vi "Answer Eval.vi"(6 "Error Deviation (%)":dbl=5.0 format="%#_13g", 7 "Exercise Number":T1, 8 "error in":errorcluster, 9 "Waveform In":waveform(dbl), 11 "Exercise Folder Path":path) -> (0 "error out":errorcluster, 1 "Waveform Out":waveform(dbl)(graph), 2 "Response Array":bool[](array[boolean]), 3 "path":path)   [LabVIEW 2014]
uses:
  Ctls/ExerciseNumeration.ctl
  <vilib>/Analysis/baseanly.llb/Mean (DBL).vi
  <vilib>/express/express analysis/Spectral/Block/exnSpectralBlock spectral measurements peak poly.vi
  <vilib>/express/express analysis/Spectral/Block/exnSpectralBlock spectral measurements peak WFM.vi
  <vilib>/express/express analysis/Spectral/XNode/ExpressSpectralMeasurementsBlockNode.xnode
  <vilib>/Analysis/NI_AAL_SigProc.lvlib
  <vilib>/Analysis/NI_AALBase.lvlib
panel:
  out "Waveform In FFT":cluster{"f0":dbl, "df":dbl, "magnitude":dbl[]}(graph)
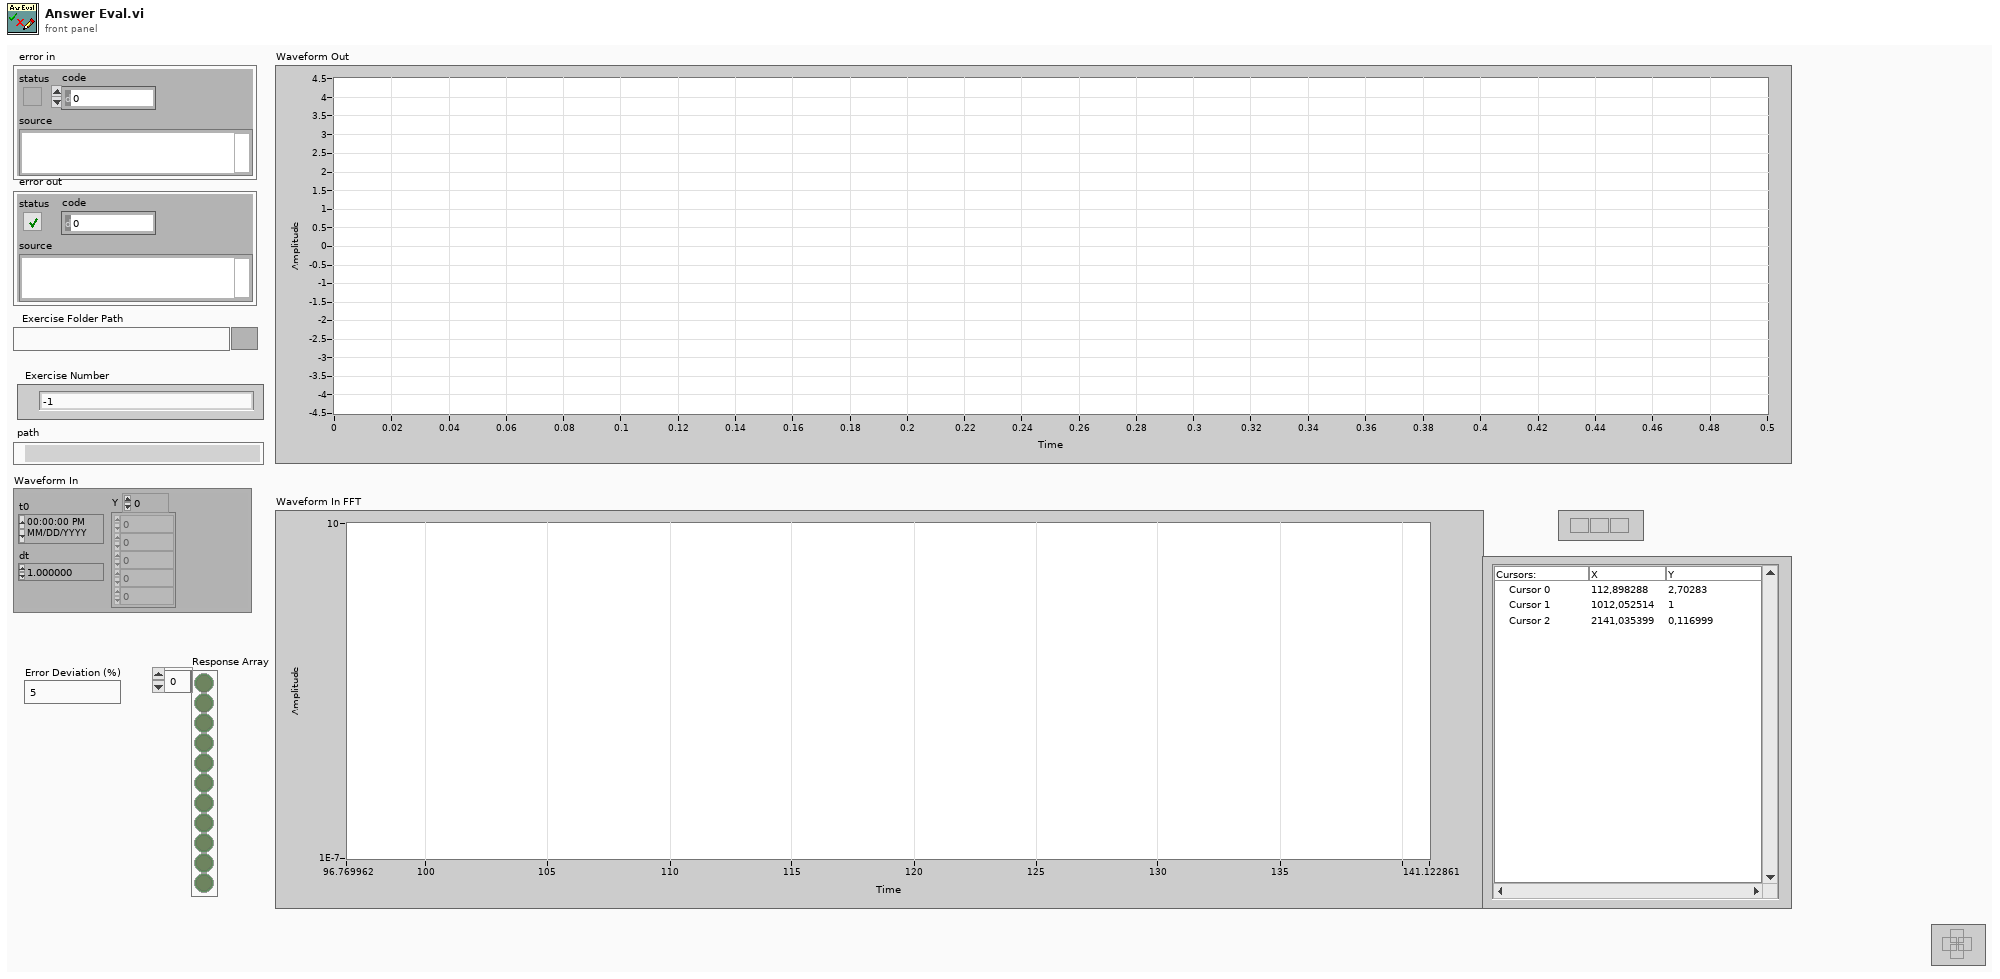
[diagram p1: front panel]
types:
  T1 = typedef "ExerciseNumeration.ctl" = enum16{"-1", "0", "1", "2", "3", "4", "5", "6", "7", "8", "9", "10"}
  T2 = enum16{"open", "replace", "create", "open or create", "replace or create", "replace or create with confirmation"}
  T3 = cluster{"averaging mode":u16, "weighting mode":u16, "number of averages":u32}
  T4 = cluster{"dB On (F)":bool, "unwrap phase (F)":bool, "convert to degree (F)":bool}
  T5 = cluster{"F1 (Hz)":dbl, "F2 (Hz)":dbl, "F3 (Hz)":dbl, "A1 (V)":dbl, "A2 (V)":dbl, "A3 (V)":dbl, "A1 (dB)":dbl, "A2 (dB)":dbl, "A3 (dB)":dbl, "Vmax (V)":dbl, "Vmin (V)":dbl, "Taxa de Aquisição (Hz)":dbl, "Resolução (bits)":dbl, "Offset (V)":dbl, "Amplificação (V/V)":dbl, "Frequência de Corte Inferior (Hz)":dbl, "Ordem do Filtro":dbl}
  T6 = cluster{"F1":dbl, "F2":dbl, "F3":dbl, "A1 (V)":dbl, "A2 (V)":dbl, "A3 (V)":dbl, "A1 (dB)":dbl, "A2 (dB)":dbl, "A3 (dB)":dbl, "Frequência de Corte\nInferior":dbl, "Ordem do \nFiltro":dbl}
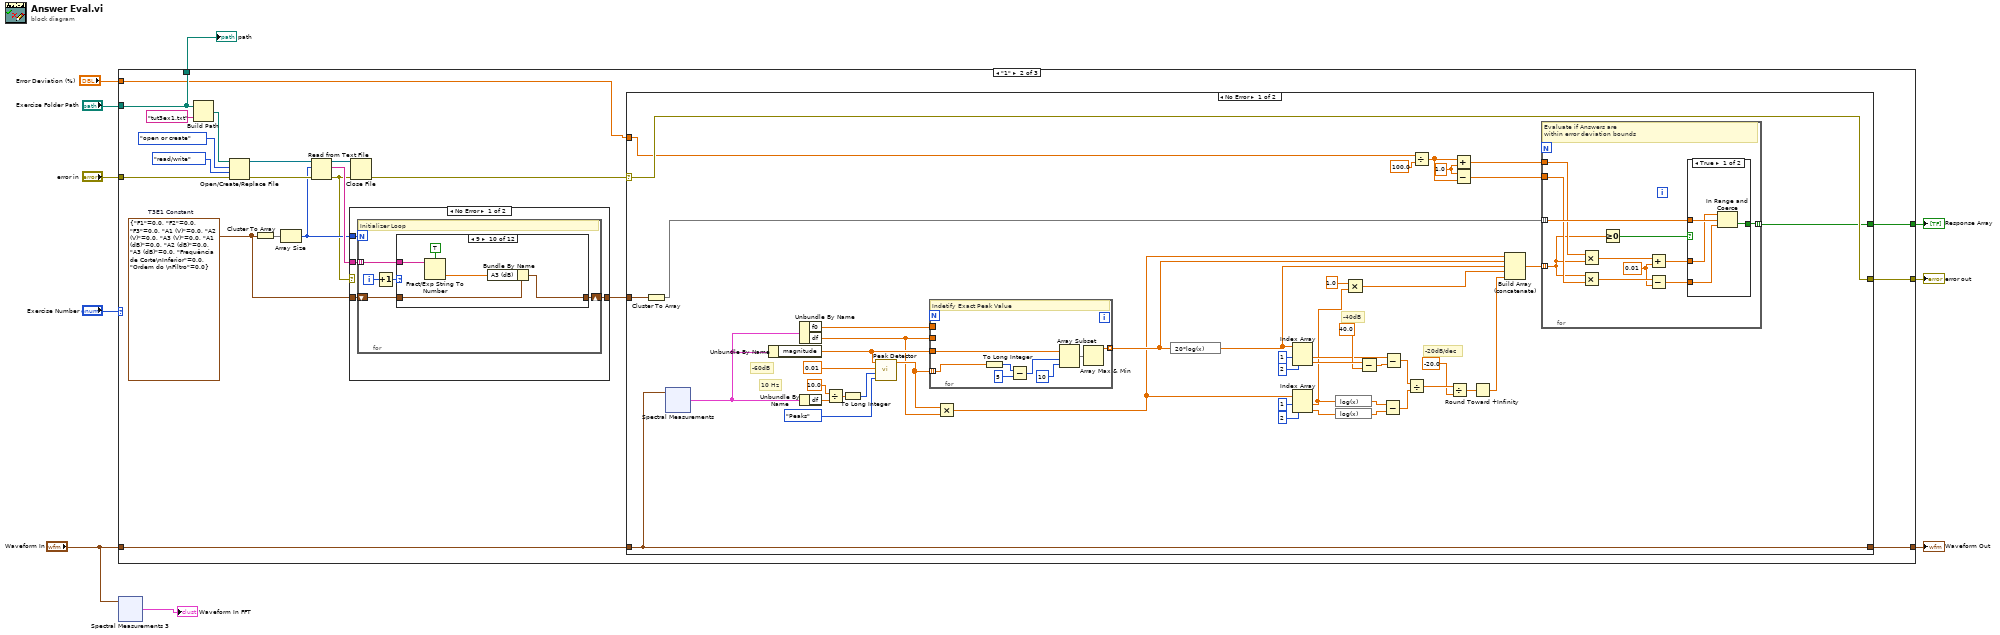
[diagram p0: block diagram]
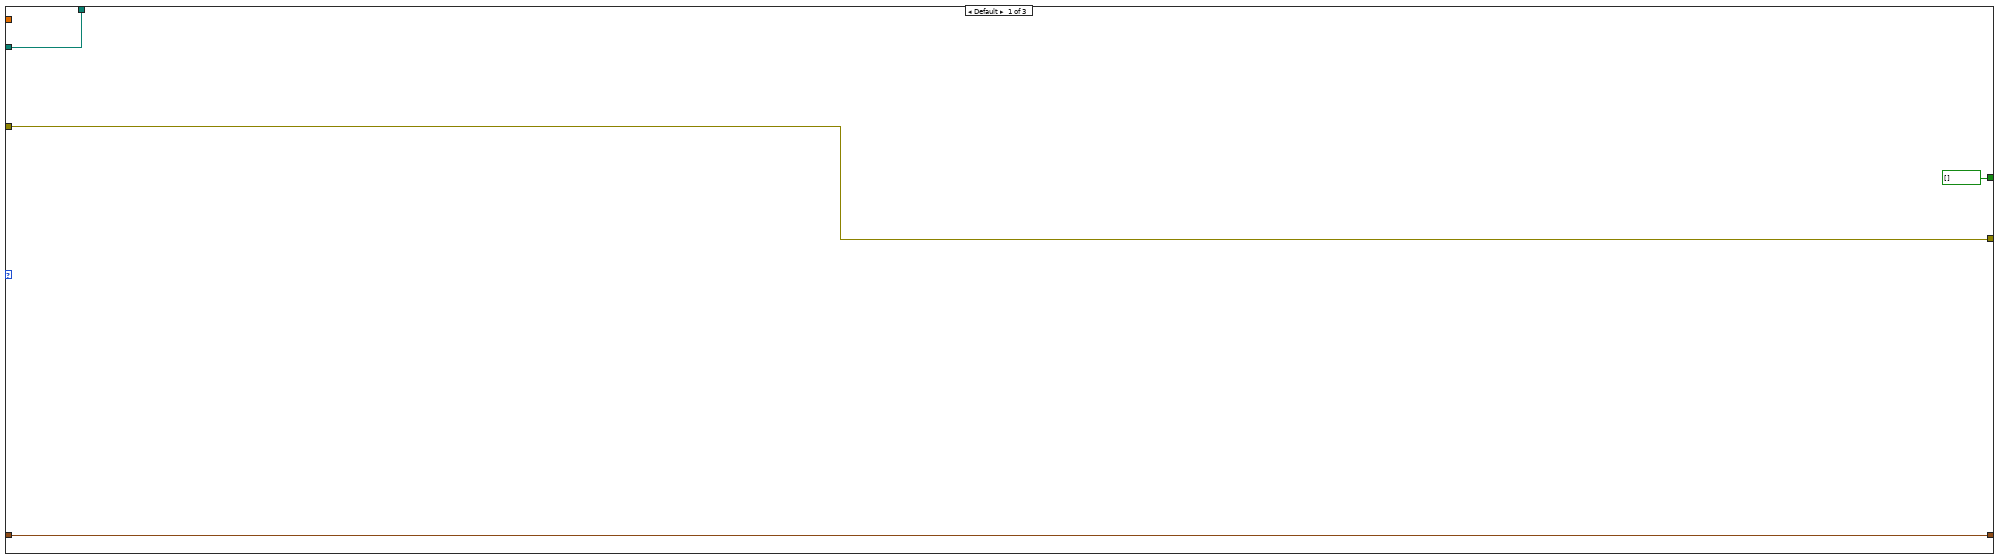
[diagram p2: hidden frame]
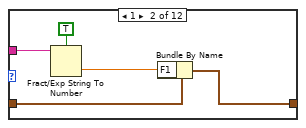
[diagram p4: hidden frame]
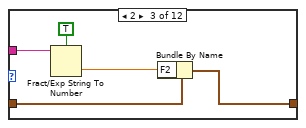
[diagram p5: hidden frame]
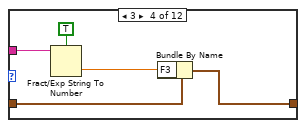
[diagram p6: hidden frame]
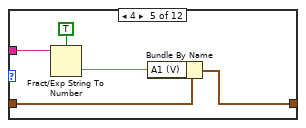
[diagram p7: hidden frame]
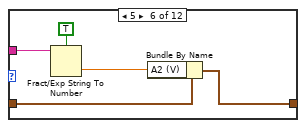
[diagram p8: hidden frame]
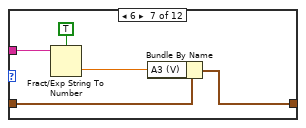
[diagram p9: hidden frame]
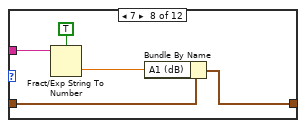
[diagram p10: hidden frame]
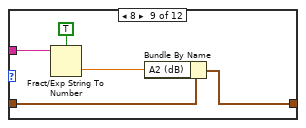
[diagram p11: hidden frame]
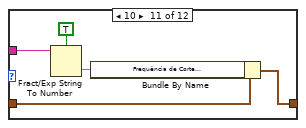
[diagram p12: hidden frame]
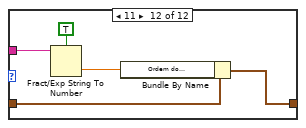
[diagram p13: hidden frame]
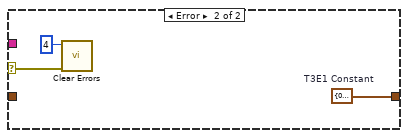
[diagram p14: hidden frame]
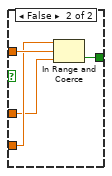
[diagram p15: hidden frame]
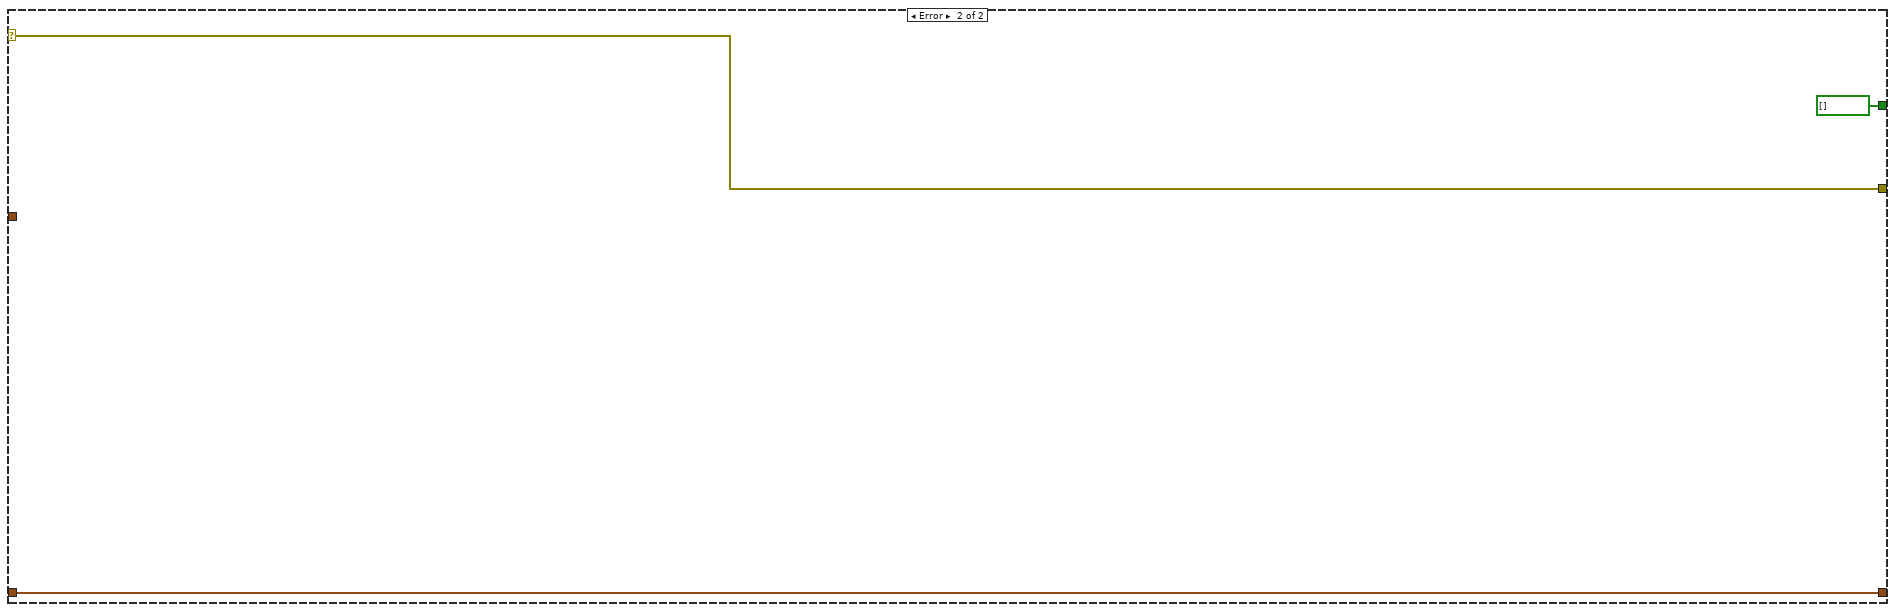
[diagram p16: hidden frame]
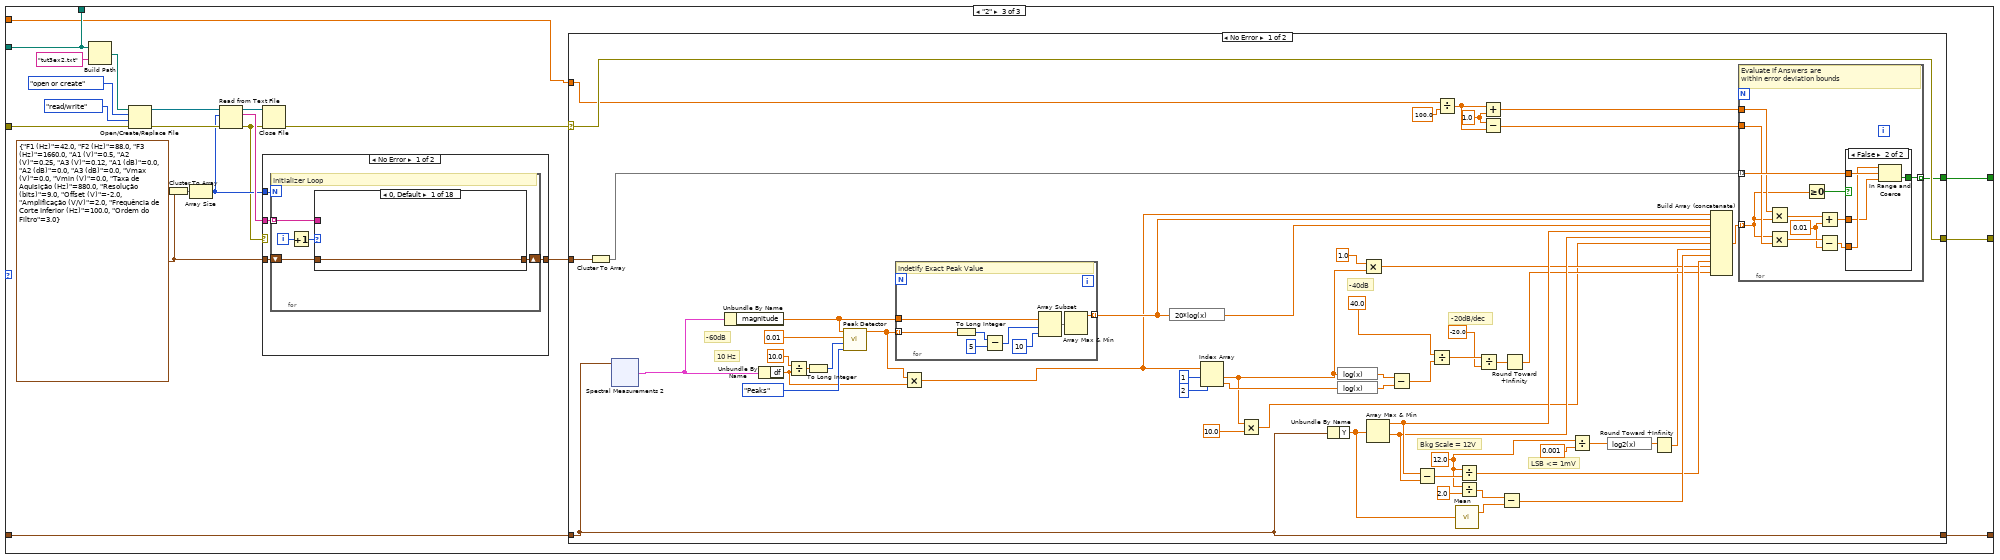
[diagram p17: hidden frame]
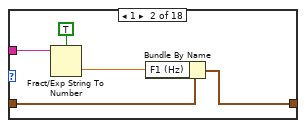
[diagram p18: hidden frame]
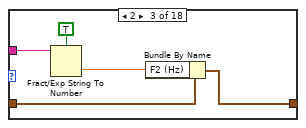
[diagram p19: hidden frame]
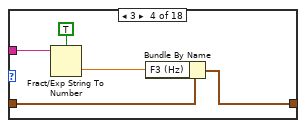
[diagram p20: hidden frame]
diagram:
  n1 = case shown="\"1\"" "Exercise Number" {
    tunnel: "Exercise Folder Path" -> [w13 w26 w201]
    tunnel: "error in" -> [w14 w33 w208]
    tunnel: [w14 w28 w203] -> w6
    tunnel: [w13 w26 w201] -> w7
    tunnel: "Waveform In" -> [w12 w18 w194]
    tunnel: [w12 w17 w193] -> w5
    tunnel: "Error Deviation (%)" -> [_ w16 w192]
    tunnel: [bool[] [] w15 w191] -> w3
    frame Default {
    }
    frame "1" {
      w23 = T6 {"F1"=0.0, "F2"=0.0, "F3"=0.0, "A1 (V)"=0.0, "A2 (V)"=0.0, "A3 (V)"=0.0, "A1 (dB)"=0.0, "A2 (dB)"=0.0, "A3 (dB)"=0.0, "Frequência de Corte\nInferior"=0.0, "Ordem do \nFiltro"=0.0}  # T3E1 Constant
      n2 = Build Path(base path=w26, name or relative path="tut3ex1.txt") -> (appended path=w34:path)
      n3 = Open/Create/Replace File(file path (use dialog)=w34, error in=w33, operation (0:open)=T2."open or create", access (0:read/write)=enum16{"read/write", "read-only", "write-only"}."read/write") -> (refnum out=w30:refnum<file>, error out=w29:errorcluster)  [unwired: 2 in, 1 out]
      n4 = Cluster To Array(cluster=w23) -> (array=w24:dbl[])
      n5 = Array Size(array=w24) -> (size(s)=w25:i32)
      n6 = Read from Text File(file (use dialog)=w30, count=w25, error in=w29) -> (refnum out=w20:refnum<file>, text=w27:string[], error out=w21:errorcluster)  [unwired: 1 in, 1 out]
      n7 = case shown="No Error" w21 {
        selector: w21 -> [_ w103]
        tunnel: w27 -> [w39 _]
        tunnel: w25 -> [w38 _]
        tunnel: w23 -> [w37 _]
        tunnel: [w36 w101] -> w22
        frame No Error {
          n8 = for {
            N: w38 -> [_]
            tunnel: w39 -> [w44] mode=indexing
            shift-right: [w40] -> w36
            shift-left: w37 -> [w41]
            i -> [w42]
            # "Initializer Loop"
            n9 = Increment(x=w42) -> (x+1=w43:i32)
            n10 = case shown="9" w43 {
              tunnel: w44 -> [_ w50 w55 w60 w65 w70 w75 w80 w85 w90 w95 w100]
              tunnel: w41 -> [w45 w48 w53 w58 w63 w68 w73 w78 w83 w88 w93 w98]
              tunnel: [w45 w46 w51 w56 w61 w66 w71 w76 w81 w86 w91 w96] -> w40
              frame 0, Default {
              }
              frame 1 {
                n11 = Fract/Exp String To Number(use system decimal point (T)=TRUE, string=w50) -> (number=w47:dbl)  [unwired: 2 in, 1 out]
                n12 = Bundle By Name(cluster=w48, "F1"=w47) -> (w46:T6)
              }
              frame 2 {
                n13 = Fract/Exp String To Number(use system decimal point (T)=TRUE, string=w55) -> (number=w52:dbl)  [unwired: 2 in, 1 out]
                n14 = Bundle By Name(cluster=w53, "F2"=w52) -> (w51:T6)
              }
              frame 3 {
                n15 = Fract/Exp String To Number(use system decimal point (T)=TRUE, string=w60) -> (number=w57:dbl)  [unwired: 2 in, 1 out]
                n16 = Bundle By Name(cluster=w58, "F3"=w57) -> (w56:T6)
              }
              frame 4 {
                n17 = Fract/Exp String To Number(use system decimal point (T)=TRUE, string=w65) -> (number=w62:dbl)  [unwired: 2 in, 1 out]
                n18 = Bundle By Name(cluster=w63, "A1 (V)"=w62) -> (w61:T6)
              }
              frame 5 {
                n19 = Fract/Exp String To Number(use system decimal point (T)=TRUE, string=w70) -> (number=w67:dbl)  [unwired: 2 in, 1 out]
                n20 = Bundle By Name(cluster=w68, "A2 (V)"=w67) -> (w66:T6)
              }
              frame 6 {
                n21 = Fract/Exp String To Number(use system decimal point (T)=TRUE, string=w75) -> (number=w72:dbl)  [unwired: 2 in, 1 out]
                n22 = Bundle By Name(cluster=w73, "A3 (V)"=w72) -> (w71:T6)
              }
              frame 7 {
                n23 = Fract/Exp String To Number(use system decimal point (T)=TRUE, string=w80) -> (number=w77:dbl)  [unwired: 2 in, 1 out]
                n24 = Bundle By Name(cluster=w78, "A1 (dB)"=w77) -> (w76:T6)
              }
              frame 8 {
                n25 = Fract/Exp String To Number(use system decimal point (T)=TRUE, string=w85) -> (number=w82:dbl)  [unwired: 2 in, 1 out]
                n26 = Bundle By Name(cluster=w83, "A2 (dB)"=w82) -> (w81:T6)
              }
              frame 9 {
                n27 = Fract/Exp String To Number(use system decimal point (T)=TRUE, string=w90) -> (number=w87:dbl)  [unwired: 2 in, 1 out]
                n28 = Bundle By Name(cluster=w88, "A3 (dB)"=w87) -> (w86:T6)
              }
              frame 10 {
                n29 = Fract/Exp String To Number(use system decimal point (T)=TRUE, string=w95) -> (number=w92:dbl)  [unwired: 2 in, 1 out]
                n30 = Bundle By Name(cluster=w93, "Frequência de Corte\nInferior"=w92) -> (w91:T6)
              }
              frame 11 {
                n31 = Fract/Exp String To Number(use system decimal point (T)=TRUE, string=w100) -> (number=w97:dbl)  [unwired: 2 in, 1 out]
                n32 = Bundle By Name(cluster=w98, "Ordem do \nFiltro"=w97) -> (w96:T6)
              }
            }
          }
        }
        frame Error {
          w101 = T6 {"F1"=0.0, "F2"=0.0, "F3"=0.0, "A1 (V)"=0.0, "A2 (V)"=0.0, "A3 (V)"=0.0, "A1 (dB)"=0.0, "A2 (dB)"=0.0, "A3 (dB)"=0.0, "Frequência de Corte\nInferior"=0.0, "Ordem do \nFiltro"=0.0}  # T3E1 Constant
          n33 = call <vilib>:"Clear Errors.vi"("error in (no error)"=w103, "specific error code to clear (0: all)"=4) -> ()  [unwired: 4 in, 2 out]
        }
      }
      n34 = Close File(refnum=w20, error in=w21) -> (error out=w19:errorcluster)  [unwired: 1 out]
      n35 = case shown="No Error" w19 {
        selector: w19 -> [w149 w189]
        tunnel: [w149 w189] -> w28
        tunnel: w22 -> [w118 _]
        tunnel: w18 -> [w143 w188]
        tunnel: [w143 w188] -> w17
        tunnel: w16 -> [w114 _]
        tunnel: [w109 bool[] []] -> w15
        frame No Error {
          w117 = 1.0 ("x")
          # "-20dB/dec"
          # "-40dB"
          # "10 Hz"
          # "-60dB"
          n36 = Cluster To Array(cluster=w118) -> (array=w112:dbl[])
          n37 = xnode "Spectral Measurements"("Signals"=w143) -> ("FFT - (Peak)"=w140:cluster{"f0":dbl, "df":dbl, "magnitude":dbl[]})  [unwired: 1 in, 2 out]
          n38 = Unbundle By Name(w140) -> ("magnitude"=w141:dbl[])
          n39 = Unbundle By Name(w140) -> ("f0"=w139:dbl, "df"=w107:dbl)
          n40 = Unbundle By Name(w140) -> ("df"=w142:dbl)
          n41 = Divide(x=10.0 ("threshold"), y=w142) -> (x/y=w146:dbl)
          n42 = To Long Integer(number=w146) -> (32bit integer=w145:i32)
          n43 = call <vilib>:"Peak Detector.vi"("peaks/valleys"=enum32{"Peaks", "Valleys"}."Peaks", "width"=w145, "threshold"=0.01, "X"=w141) -> ("Locations"=w108:dbl[])  [unwired: 3 in, 4 out]
          n44 = for {
            tunnel: w108 -> [w169] mode=indexing
            tunnel: w141 -> [w174]
            tunnel: w107 -> [_]
            tunnel: w139 -> [_]
            tunnel: [w170] -> w124 mode=indexing
            # "Indetify Exact Peak Value"
            n45 = To Long Integer(number=w169) -> (32bit integer=w176:i32)
            n46 = Subtract(x=w176, y=5) -> (x-y=w173:i32)
            n47 = Array Subset(array=w174, index=w173, length=10) -> (w171:dbl[])
            n48 = Array Max & Min(array=w171) -> (max value=w170:dbl)  [unwired: 3 out]
          }
          n49 = Multiply(x=w108, y=w107) -> (x*y=w106:dbl[])
          n50 = expression code="20*log(x)"(w124) -> (w123:dbl[])
          n51 = Index Array(array=w123, index #1=1 ("index"), index #2=2 ("index")) -> (element #1=w131:dbl, element #2=w134:dbl)
          n52 = Index Array(array=w106, index #1=1 ("index"), index #2=2 ("index")) -> (element #1=w104:dbl, element #2=w105:dbl)
          n53 = expression code="log(x)"(w104) -> (w126:dbl)
          n54 = expression code="log(x)"(w105) -> (w125:dbl)
          n55 = Multiply(x=1.0, y=w104) -> (x*y=w121:dbl)
          n56 = Subtract(x=w134, y=40.0) -> (x-y=w132:dbl)
          n57 = Subtract(x=w126, y=w125) -> (x-y=w129:dbl)
          n58 = Subtract(x=w131, y=w132) -> (x-y=w130:dbl)
          n59 = Divide(x=w130, y=w129) -> (x/y=w128:dbl)
          n60 = Divide(x=w114, y=100.0) -> (x/y=w115:dbl)
          n61 = Divide(x=w128, y=-20.0) -> (x/y=w120:dbl)
          n62 = Add(x=w115, y=w117) -> (x+y=w110:dbl)
          n63 = Subtract(x=w117, y=w115) -> (x-y=w111:dbl)
          n64 = Round Toward +Infinity(x=w120) -> (ceil(x): smallest int >= x=w119:dbl)
          n65 = Build Array (concatenate)(w106, w124, w123, w121, w119) -> (w113:dbl[])
          n66 = for {
            tunnel: w113 -> [w155] mode=indexing
            tunnel: w112 -> [w160] mode=indexing
            tunnel: w110 -> [w159]
            tunnel: w111 -> [w158]
            tunnel: [w157] -> w109 mode=indexing
            w150 = 0.01 ("x")
            # "Evaluate if Answers are\nwithin error deviation bounds"
            n67 = Multiply(x=w159, y=w155) -> (x*y=w154:dbl)
            n68 = Multiply(x=w155, y=w158) -> (x*y=w151:dbl)
            n69 = Greater Or Equal To 0?(x=w155) -> (x >= 0?=w156:bool)
            n70 = Add(x=w154, y=w150) -> (x+y=w152:dbl)
            n71 = Subtract(x=w151, y=w150) -> (x-y=w153:dbl)
            n72 = case shown="True" w156 {
              tunnel: w160 -> [w164 w168]
              tunnel: w152 -> [w163 w165]
              tunnel: w153 -> [w162 w166]
              tunnel: [w161 w167] -> w157
              frame True {
                n73 = In Range and Coerce(upper limit=w163, x=w164, lower limit=w162) -> (In Range?=w161:bool)  [unwired: 1 out]
              }
              frame False {
                n74 = In Range and Coerce(upper limit=w166, x=w168, lower limit=w165) -> (In Range?=w167:bool)  [unwired: 1 out]
              }
            }
          }
        }
        frame Error {
        }
      }
    }
    frame "2" {
      w190 = T5 {"F1 (Hz)"=42.0, "F2 (Hz)"=88.0, "F3 (Hz)"=1660.0, "A1 (V)"=0.5, "A2 (V)"=0.25, "A3 (V)"=0.12, "A1 (dB)"=0.0, "A2 (dB)"=0.0, "A3 (dB)"=0.0, "Vmax (V)"=0.0, "Vmin (V)"=0.0, "Taxa de Aquisição (Hz)"=880.0, "Resolução (bits)"=9.0, "Offset (V)"=-2.0, "Amplificação (V/V)"=2.0, "Frequência de Corte Inferior (Hz)"=100.0, "Ordem do Filtro"=3.0} ("T3E2")
      n75 = Build Path(base path=w201, name or relative path="tut3ex2.txt") -> (appended path=w209:path)
      n76 = Open/Create/Replace File(file path (use dialog)=w209, error in=w208, operation (0:open)=T2."open or create", access (0:read/write)=enum16{"read/write", "read-only", "write-only"}."read/write") -> (refnum out=w205:refnum<file>, error out=w204:errorcluster)  [unwired: 2 in, 1 out]
      n77 = Cluster To Array(cluster=w190) -> (array=w199:dbl[])
      n78 = Array Size(array=w199) -> (size(s)=w200:i32)
      n79 = Read from Text File(file (use dialog)=w205, count=w200, error in=w204) -> (refnum out=w196:refnum<file>, text=w202:string[], error out=w197:errorcluster)  [unwired: 1 in, 1 out]
      n80 = case shown="No Error" w197 {
        selector: w197 -> [_ w308]
        tunnel: w202 -> [w214 _]
        tunnel: w200 -> [w213 _]
        tunnel: [w211 T5 {"F1 (Hz)"=0.0, "F2 (Hz)"=0.0, "F3 (Hz)"=0.0, "A1 (V)"=0.0, "A2 (V)"=0.0, "A3 (V)"=0.0, "A1 (dB)"=0.0, "A2 (dB)"=0.0, "A3 (dB)"=0.0, "Vmax (V)"=0.0, "Vmin (V)"=0.0, "Taxa de Aquisição (Hz)"=0.0, "Resolução (bits)"=0.0, "Offset (V)"=0.0, "Amplificação (V/V)"=0.0, "Frequência de Corte Inferior (Hz)"=0.0, "Ordem do Filtro"=0.0} ("T3E2")] -> w198
        tunnel: w190 -> [w212 _]
        frame No Error {
          n81 = for {
            N: w213 -> [_]
            tunnel: w214 -> [w219] mode=indexing
            shift-right: [w215] -> w211
            shift-left: w212 -> [w216]
            i -> [w217]
            # "Initializer Loop"
            n82 = Increment(x=w217) -> (x+1=w218:i32)
            n83 = case shown="0, Default" w218 {
              tunnel: w219 -> [_ w225 w230 w235 w240 w245 w250 w255 w260 w265 w270 w275 w280 w285 w290 w295 w300 w305]
              tunnel: w216 -> [w220 w223 w228 w233 w238 w243 w248 w253 w258 w263 w268 w273 w278 w283 w288 w293 w298 w303]
              tunnel: [w220 w221 w226 w231 w236 w241 w246 w251 w256 w261 w266 w271 w276 w281 w286 w291 w296 w301] -> w215
              frame 0, Default {
              }
              frame 1 {
                n84 = Fract/Exp String To Number(use system decimal point (T)=TRUE, string=w225) -> (number=w222:dbl)  [unwired: 2 in, 1 out]
                n85 = Bundle By Name(cluster=w223, "F1 (Hz)"=w222) -> (w221:T5)
              }
              frame 2 {
                n86 = Fract/Exp String To Number(use system decimal point (T)=TRUE, string=w230) -> (number=w227:dbl)  [unwired: 2 in, 1 out]
                n87 = Bundle By Name(cluster=w228, "F2 (Hz)"=w227) -> (w226:T5)
              }
              frame 3 {
                n88 = Fract/Exp String To Number(use system decimal point (T)=TRUE, string=w235) -> (number=w232:dbl)  [unwired: 2 in, 1 out]
                n89 = Bundle By Name(cluster=w233, "F3 (Hz)"=w232) -> (w231:T5)
              }
              frame 4 {
                n90 = Fract/Exp String To Number(use system decimal point (T)=TRUE, string=w240) -> (number=w237:dbl)  [unwired: 2 in, 1 out]
                n91 = Bundle By Name(cluster=w238, "A1 (V)"=w237) -> (w236:T5)
              }
              frame 5 {
                n92 = Fract/Exp String To Number(use system decimal point (T)=TRUE, string=w245) -> (number=w242:dbl)  [unwired: 2 in, 1 out]
                n93 = Bundle By Name(cluster=w243, "A2 (V)"=w242) -> (w241:T5)
              }
              frame 6 {
                n94 = Fract/Exp String To Number(use system decimal point (T)=TRUE, string=w250) -> (number=w247:dbl)  [unwired: 2 in, 1 out]
                n95 = Bundle By Name(cluster=w248, "A3 (V)"=w247) -> (w246:T5)
              }
              frame 7 {
                n96 = Fract/Exp String To Number(use system decimal point (T)=TRUE, string=w255) -> (number=w252:dbl)  [unwired: 2 in, 1 out]
                n97 = Bundle By Name(cluster=w253, "A1 (dB)"=w252) -> (w251:T5)
              }
              frame 8 {
                n98 = Fract/Exp String To Number(use system decimal point (T)=TRUE, string=w260) -> (number=w257:dbl)  [unwired: 2 in, 1 out]
                n99 = Bundle By Name(cluster=w258, "A2 (dB)"=w257) -> (w256:T5)
              }
              frame 9 {
                n100 = Fract/Exp String To Number(use system decimal point (T)=TRUE, string=w265) -> (number=w262:dbl)  [unwired: 2 in, 1 out]
                n101 = Bundle By Name(cluster=w263, "A3 (dB)"=w262) -> (w261:T5)
              }
              frame 10 {
                n102 = Fract/Exp String To Number(use system decimal point (T)=TRUE, string=w270) -> (number=w267:dbl)  [unwired: 2 in, 1 out]
                n103 = Bundle By Name(cluster=w268, "Vmax (V)"=w267) -> (w266:T5)
              }
              frame 11 {
                n104 = Fract/Exp String To Number(use system decimal point (T)=TRUE, string=w275) -> (number=w272:dbl)  [unwired: 2 in, 1 out]
                n105 = Bundle By Name(cluster=w273, "Vmin (V)"=w272) -> (w271:T5)
              }
              frame 12 {
                n106 = Fract/Exp String To Number(use system decimal point (T)=TRUE, string=w280) -> (number=w277:dbl)  [unwired: 2 in, 1 out]
                n107 = Bundle By Name(cluster=w278, "Taxa de Aquisição (Hz)"=w277) -> (w276:T5)
              }
              frame 13 {
                n108 = Fract/Exp String To Number(use system decimal point (T)=TRUE, string=w285) -> (number=w282:dbl)  [unwired: 2 in, 1 out]
                n109 = Bundle By Name(cluster=w283, "Resolução (bits)"=w282) -> (w281:T5)
              }
              frame 14 {
                n110 = Fract/Exp String To Number(use system decimal point (T)=TRUE, string=w290) -> (number=w287:dbl)  [unwired: 2 in, 1 out]
                n111 = Bundle By Name(cluster=w288, "Offset (V)"=w287) -> (w286:T5)
              }
              frame 15 {
                n112 = Fract/Exp String To Number(use system decimal point (T)=TRUE, string=w295) -> (number=w292:dbl)  [unwired: 2 in, 1 out]
                n113 = Bundle By Name(cluster=w293, "Amplificação (V/V)"=w292) -> (w291:T5)
              }
              frame 16 {
                n114 = Fract/Exp String To Number(use system decimal point (T)=TRUE, string=w300) -> (number=w297:dbl)  [unwired: 2 in, 1 out]
                n115 = Bundle By Name(cluster=w298, "Frequência de Corte Inferior (Hz)"=w297) -> (w296:T5)
              }
              frame 17 {
                n116 = Fract/Exp String To Number(use system decimal point (T)=TRUE, string=w305) -> (number=w302:dbl)  [unwired: 2 in, 1 out]
                n117 = Bundle By Name(cluster=w303, "Ordem do Filtro"=w302) -> (w301:T5)
              }
            }
          }
        }
        frame Error {
          n118 = call <vilib>:"Clear Errors.vi"("error in (no error)"=w308, "specific error code to clear (0: all)"=4) -> ()  [unwired: 4 in, 2 out]
        }
      }
      n119 = Close File(refnum=w196, error in=w197) -> (error out=w195:errorcluster)  [unwired: 1 out]
      n120 = case shown="No Error" w195 {
        selector: w195 -> [w362 w402]
        tunnel: [w362 w402] -> w203
        tunnel: w198 -> [w346 _]
        tunnel: w194 -> [w337 w401]
        tunnel: [w337 w401] -> w193
        tunnel: w192 -> [w341 _]
        tunnel: [w338 bool[] []] -> w191
        frame No Error {
          w325 = 12.0 ("y")
          w344 = 1.0 ("x")
          # "Bkg Scale = 12V"
          # "LSB <= 1mV"
          # "-20dB/dec"
          # "-40dB"
          # "10 Hz"
          # "-60dB"
          n121 = Cluster To Array(cluster=w346) -> (array=w345:dbl[])
          n122 = xnode "Spectral Measurements 2"("Signals"=w337) -> ("FFT - (Peak)"=w356:cluster{"f0":dbl, "df":dbl, "magnitude":dbl[]})  [unwired: 1 in, 2 out]
          n123 = Unbundle By Name(w356) -> ("magnitude"=w320:dbl[])
          n124 = Unbundle By Name(w356) -> ("df"=w317:dbl)
          n125 = Divide(x=10.0 ("threshold"), y=w317) -> (x/y=w359:dbl)
          n126 = To Long Integer(number=w359) -> (32bit integer=w358:i32)
          n127 = call <vilib>:"Peak Detector.vi"("peaks/valleys"=enum32{"Peaks", "Valleys"}."Peaks", "width"=w358, "threshold"=0.01, "X"=w320) -> ("Locations"=w318:dbl[])  [unwired: 3 in, 4 out]
          n128 = for {
            tunnel: w318 -> [w363] mode=indexing
            tunnel: w320 -> [w368]
            tunnel: [w364] -> w319 mode=indexing
            # "Indetify Exact Peak Value"
            n129 = To Long Integer(number=w363) -> (32bit integer=w370:i32)
            n130 = Subtract(x=w370, y=5) -> (x-y=w367:i32)
            n131 = Array Subset(array=w368, index=w367, length=10) -> (w365:dbl[])
            n132 = Array Max & Min(array=w365) -> (max value=w364:dbl)  [unwired: 3 out]
          }
          n133 = Multiply(x=w318, y=w317) -> (x*y=w315:dbl[])
          n134 = expression code="20*log(x)"(w319) -> (w350:dbl[])
          n135 = Index Array(array=w315, index #1=1 ("index"), index #2=2 ("index")) -> (element #1=w311:dbl, element #2=w312:dbl)
          n136 = Multiply(x=w311, y=10.0) -> (x*y=w309:dbl)
          n137 = Unbundle By Name(w337) -> ("Y"=w333:dbl[])
          n138 = expression code="log(x)"(w311) -> (w352:dbl)
          n139 = expression code="log(x)"(w312) -> (w351:dbl)
          n140 = Multiply(x=1.0, y=w311) -> (x*y=w327:dbl)
          n141 = Array Max & Min(array=w333) -> (max value=w336:dbl, min value=w335:dbl)  [unwired: 2 out]
          n142 = Subtract(x=w352, y=w351) -> (x-y=w355:dbl)
          n143 = Subtract(x=w336, y=w335) -> (x-y=w334:dbl)
          n144 = Divide(x=40.0 ("y"), y=w355) -> (x/y=w354:dbl)
          n145 = Divide(x=w341, y=100.0) -> (x/y=w342:dbl)
          n146 = call-poly <vilib>:"Mean.vi"("X"=w333) -> ("mean"=w330:dbl)  [unwired: 1 out]
          n147 = Divide(x=w325, y=w334) -> (x/y=w328:dbl)
          n148 = Divide(x=w325, y=2.0) -> (x/y=w331:dbl)
          n149 = Divide(x=w354, y=-20.0) -> (x/y=w348:dbl)
          n150 = Add(x=w342, y=w344) -> (x+y=w340:dbl)
          n151 = Subtract(x=w344, y=w342) -> (x-y=w339:dbl)
          n152 = Subtract(x=w331, y=w330) -> (x-y=w329:dbl)
          n153 = Round Toward +Infinity(x=w348) -> (ceil(x): smallest int >= x=w326:dbl)
          n154 = Divide(x=w325, y=0.001) -> (x/y=w323:dbl)
          n155 = expression code="log2(x)"(w323) -> (w322:dbl)
          n156 = Round Toward +Infinity(x=w322) -> (ceil(x): smallest int >= x=w321:dbl)
          n157 = Build Array (concatenate)(w315, w319, w350, w336, w335, w309, w321, w329, w328, w327, w326) -> (w347:dbl[])
          n158 = for {
            tunnel: w347 -> [w376] mode=indexing
            tunnel: w345 -> [w381] mode=indexing
            tunnel: w340 -> [w380]
            tunnel: w339 -> [w379]
            tunnel: [w378] -> w338 mode=indexing
            w371 = 0.01 ("x")
            # "Evaluate if Answers are\nwithin error deviation bounds"
            n159 = Multiply(x=w380, y=w376) -> (x*y=w375:dbl)
            n160 = Multiply(x=w376, y=w379) -> (x*y=w372:dbl)
            n161 = Greater Or Equal To 0?(x=w376) -> (x >= 0?=w377:bool)
            n162 = Add(x=w375, y=w371) -> (x+y=w373:dbl)
            n163 = Subtract(x=w372, y=w371) -> (x-y=w374:dbl)
            n164 = case shown="False" w377 {
              tunnel: w381 -> [w385 w389]
              tunnel: w373 -> [w384 w386]
              tunnel: w374 -> [w383 w387]
              tunnel: [w382 w388] -> w378
              frame True {
                n165 = In Range and Coerce(upper limit=w384, x=w385, lower limit=w383) -> (In Range?=w382:bool)  [unwired: 1 out]
              }
              frame False {
                n166 = In Range and Coerce(upper limit=w387, x=w389, lower limit=w386) -> (In Range?=w388:bool)  [unwired: 1 out]
              }
            }
          }
        }
        frame Error {
        }
      }
    }
  }
  "error out" <- w6
  "path" <- w7
  "Waveform Out" <- w5
  "Response Array" <- w3
  n167 = xnode "Spectral Measurements 3"("Signals"="Waveform In") -> ("FFT - (Peak)"=→"Waveform In FFT":cluster{"f0":dbl, "df":dbl, "magnitude":dbl[]})  [unwired: 1 in, 2 out]
